vi "Format Word for CSV.vi"(8 "error in":errorcluster, 10 "data word format":T1="Hexadecimal", 11 "word":T2 {"type" format="%04x"; "activity" format="%04x"; "error" format="%04x"; "cwd1" format="%04x"; "cwd2" format="%04x"; "swd1" format="%04x"; "swd2" format="%04x"; "data" format="%04x"}) -> (0 "error out":errorcluster, 3 "string":string[](array[string]))   [LabVIEW 2020, in "AIM MIL-STD-1553 Engine.lvlib" / "Implementation.lvlib" / "CSV Word Logger.lvclass"]
uses:
  CSV Word Logger.lvclass
  Word.ctl
  Shared/Data Word Format.ctl
  Rx Execution Unit/Rx Execution Unit.lvclass
  <instrlib>/BTI1553Lib/BTI1553LV.lvlib
  Implementation.lvlib
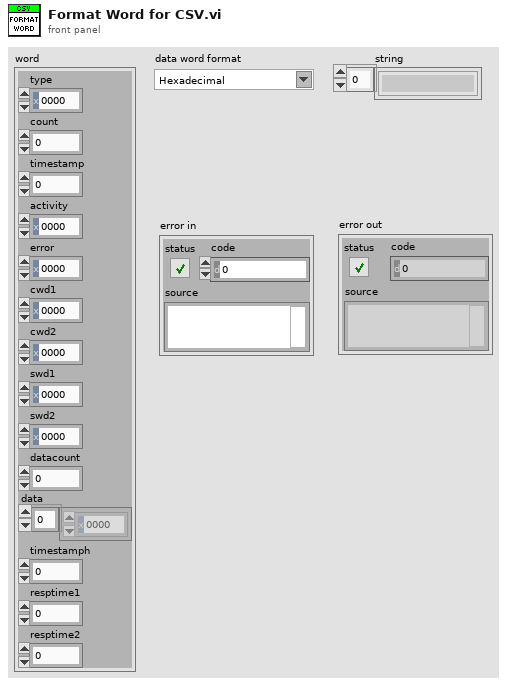
[diagram p1: front panel]
types:
  T1 = typedef "Data Word Format.ctl" = string
  T2 = typedef "AIM MIL-STD-1553 Engine.lvlib/Implementation.lvlib/Word.ctl" = cluster{"type":u16, "count":u16, "timestamp":u32, "activity":u16, "error":u16, "cwd1":u16, "cwd2":u16, "swd1":u16, "swd2":u16, "datacount":u16, "data":u16[], "timestamph":u32, "resptime1":u16, "resptime2":u16}
  T3 = typedef "BTI1553LV.lvlib/1553 Activity Flags.ctl" = cluster{"channelnumber":i32, "transmittedcwd1":bool, "transmittedcwd2":bool, "transmittedswd1":bool, "transmittedswd2":bool, "receivedcwd1":bool, "receivedcwd2":bool, "receivedswd1":bool, "receivedswd2":bool, "transmitteddwd":bool, "receiveddwd":bool, "reserved1":i8, "reserved2":i8, "bus":u32}
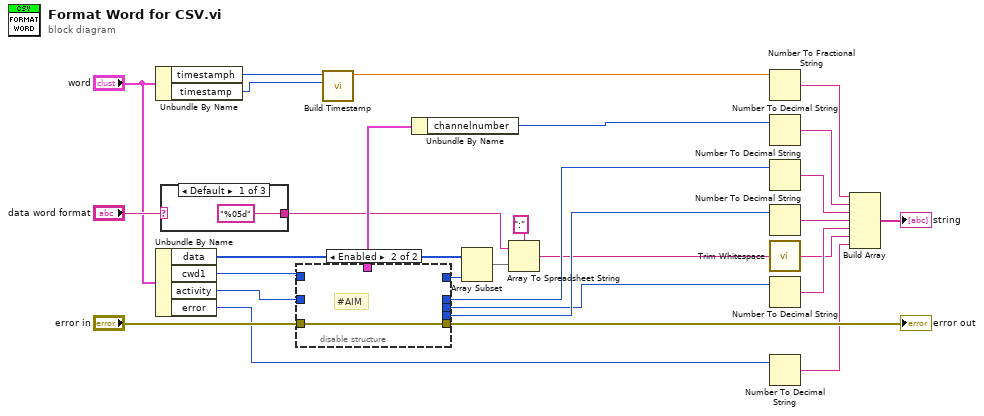
[diagram p0: block diagram]
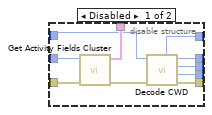
[diagram p2: hidden frame]
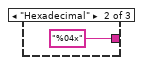
[diagram p3: hidden frame]
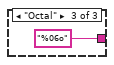
[diagram p4: hidden frame]
diagram:
  n1 = Unbundle By Name("word") -> ("timestamph"=w4:u32, "timestamp"=w3:u32)
  n2 = Unbundle By Name("word") -> ("data"=w1:u16[], "cwd1"=w18:u16, "activity"=w22:u16, "error"=w2:u16)
  n3 = case shown="Default" "data word format" {
    tunnel: ["%05d" ("format string") "%04x" ("format string") "%06o" ("format string")] -> w13
    frame Default {
    }
    frame "Hexadecimal" {
    }
    frame "Octal" {
    }
  }
  n4 = disable-structure shown="Enabled" {
    disable-tunnel: w22 -> [w42 _]
    disable-tunnel: [w41 _] -> w21
    disable-tunnel: "error in" -> [w40 w43]
    disable-tunnel: w18 -> [w38 _]
    disable-tunnel: [w37 _] -> w17
    disable-tunnel: [w36 _] -> w16
    disable-tunnel: [w35 _] -> w15
    disable-tunnel: [w34 w43] -> w11
    disable-tunnel: [w33 _] -> w9
    frame Disabled {
      n5 = call <instrlib>:"Get Activity Fields Cluster.vi"("error in (no error)"=w40, "activity"=w42) -> ("error out"=w39:errorcluster, "activity flags"=w41:T3)  [unwired: 8 in]
      n6 = call <instrlib>:"Decode CWD.vi"("error in (no error)"=w39, "command word"=w38) -> ("error out"=w34:errorcluster, "subaddress out"=w36:i32, "transmit/receive bit value out"=w35:i32, "terminal address out"=w37:i32, "word count out"=w33:i32)  [unwired: 5 in]
    }
    frame Enabled {
      # "#AIM"
    }
  }
  "error out" <- w11
  n7 = call "Build Timestamp.vi"("timestamp low bits"=w3, "timestamp high bits"=w4) -> ("timestamp out"=w23:dbl)  [unwired: 9 in]
  n8 = Unbundle By Name(w21) -> ("channelnumber"=w20:i32)
  n9 = Array Subset(array=w1, length=w9) -> (w10:u16[])  [unwired: 1 in]
  n10 = Array To Spreadsheet String(delimiter (Tab)=":", array=w10, 3:w13) -> (spreadsheet string=w7:string)
  n11 = Number To Fractional String(number=w23) -> (F-format string=w28:string)  [unwired: 3 in]
  n12 = Number To Decimal String(number=w20) -> (decimal integer string=w25:string)  [unwired: 1 in]
  n13 = Number To Decimal String(number=w17) -> (decimal integer string=w27:string)  [unwired: 1 in]
  n14 = Number To Decimal String(number=w16) -> (decimal integer string=w26:string)  [unwired: 1 in]
  n15 = call <vilib>:"Trim Whitespace.vi"("string"=w7) -> ("trimmed string"=w6:string)  [unwired: 1 in]
  n16 = Number To Decimal String(number=w15) -> (decimal integer string=w12:string)  [unwired: 1 in]
  n17 = Number To Decimal String(number=w2) -> (decimal integer string=w8:string)  [unwired: 1 in]
  n18 = Build Array(w28, w25, w27, w26, w12, w6, w8) -> (→"string":string[])
